vi "define_stimulus_shape.vi"(8 "error in":errorcluster, 10 "input cluster":T1={"base directory"=path "", "data directory"=path "", "active"=FALSE, "running"=FALSE, "pairing"=FALSE, "clean tubes"=FALSE, "animal ID"=0, "session ID"=0, "base temp"=0.0, "d wait min"=0, "d wait max"=0, "d timeout"=0, "d reward"=0, "idx stim"=0, "timeout win"=0, "lick win"=[], "stim type"=[], "stim dur"=[], "stim amp"=[], "stim freq"=[], "stim ramp"=[], "stim catch"=[], "square dur"=[50, 20, 10], "square delay"=[50, 20, 10], "square freq"=[], "square dc"=[50, 20, 10], "stim shape"=[], "square shape"=[]} {"stim ramp" min=1}) -> (0 "error out":errorcluster, 2 "output cluster":T1={"base directory"=path "", "data directory"=path "", "active"=FALSE, "running"=FALSE, "pairing"=FALSE, "clean tubes"=FALSE, "animal ID"=0, "session ID"=0, "base temp"=0.0, "d wait min"=0, "d wait max"=0, "d timeout"=0, "d reward"=0, "idx stim"=0, "timeout win"=0, "lick win"=[], "stim type"=[enum."sine", enum."square", enum."pulse"], "stim dur"=[500, 500, 1000], "stim amp"=[1.0, 1.0, 1.0], "stim freq"=[20, 20, 20], "stim ramp"=[100, 200, 200], "stim catch"=[], "square dur"=[50, 20, 10], "square delay"=[50, 20, 10], "square freq"=[], "square dc"=[50, 20, 10], "stim shape"=array3x1000[3000 elements], "square shape"=[]} {"stim ramp" min=1})   [LabVIEW 2016]
uses:
  Type Definitions/vars_settings.ctl
  Type Definitions/stim_type.ctl
  <vilib>/Analysis/1siggen.llb/Ramp Pattern.vi
  <vilib>/Analysis/1siggen.llb/Ramp Pattern by Samples.vi
  <vilib>/Utility/error.llb/Error Cluster From Error Code.vi
  <vilib>/Analysis/NI_AALBase.lvlib
panel:
  out "stim shape":dbl[][](graph)
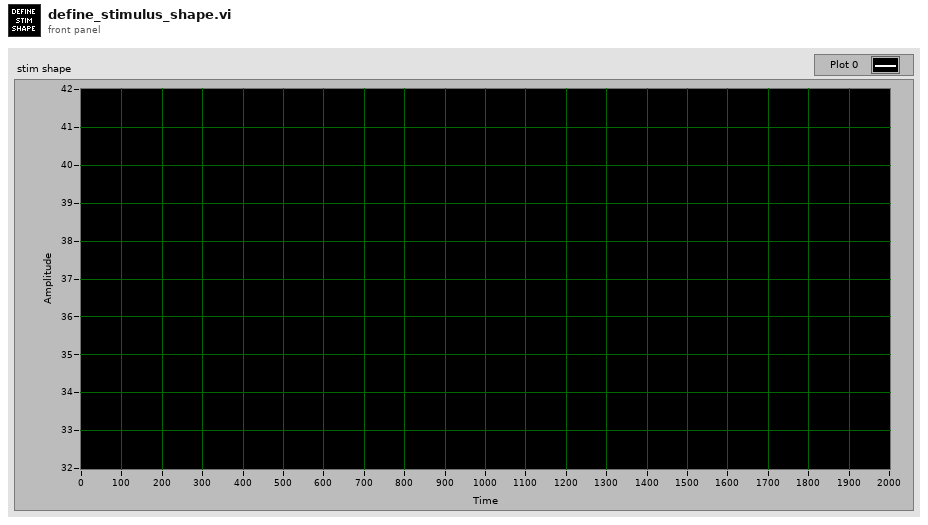
[diagram p1: front panel]
types:
  T1 = typedef "vars_settings.ctl" = cluster{"base directory":path, "data directory":path, "active":bool, "running":bool, "pairing":bool, "clean tubes":bool, "animal ID":u16, "session ID":u16, "base temp":dbl, "d wait min":u16, "d wait max":u16, "d timeout":u16, "d reward":u16, "idx stim":u16, "timeout win":u16, "lick win":i32[], "stim type":T2[], "stim dur":u16[], "stim amp":dbl[], "stim freq":u16[], "stim ramp":u16[], "stim catch":u8[], "square dur":u8[], "square delay":u8[], "square freq":u8[], "square dc":u8[], "stim shape":dbl[][], "square shape":bool[][]}
  T2 = typedef "stim_type.ctl" = enum16{"pulse", "vibration", "square", "sine"}
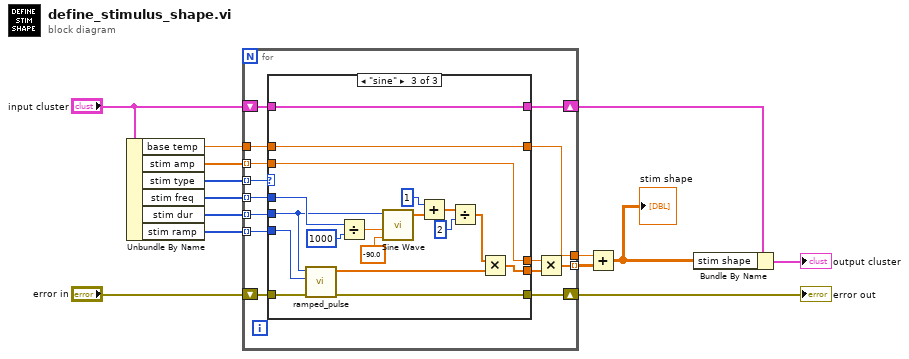
[diagram p0: block diagram]
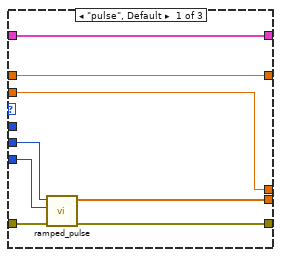
[diagram p2: hidden frame]
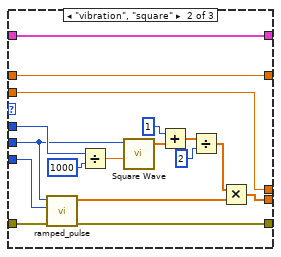
[diagram p3: hidden frame]
diagram:
  n1 = Unbundle By Name("input cluster") -> ("base temp"=w4:dbl, "stim amp"=w5:dbl[], "stim type"=w11:T2[], "stim freq"=w8:u16[], "stim dur"=w6:u16[], "stim ramp"=w7:u16[])
  n2 = for {
    tunnel: w11 -> [w25] mode=indexing
    shift-right: [w28] -> w14
    shift-left: "error in" -> [w27]
    shift-right: [w24] -> w9
    shift-left: "input cluster" -> [w26]
    tunnel: w8 -> [w23] mode=indexing
    tunnel: w6 -> [w22] mode=indexing
    tunnel: w7 -> [w21] mode=indexing
    tunnel: w5 -> [w20] mode=indexing
    tunnel: w4 -> [w19]
    tunnel: [w16] -> w3 mode=indexing
    tunnel: [w15] -> w2
    n3 = case shown="\"sine\"" w25 {
      tunnel: [w36 w53 w71] -> w28
      tunnel: w27 -> [w35 w52 w70]
      tunnel: w26 -> [w34 w51 w69]
      tunnel: [w34 w51 w69] -> w24
      tunnel: [w29 w42 w62] -> w18
      tunnel: w22 -> [w30 w40 w57]
      tunnel: w21 -> [w33 w39 w56]
      tunnel: w23 -> [_ w41 w58]
      tunnel: w20 -> [w32 w37 w54]
      tunnel: [w32 w37 w54] -> w17
      tunnel: [w31 w38 w55] -> w15
      tunnel: w19 -> [w31 w38 w55]
      frame "pulse", Default {
        n4 = call "ramped_pulse.vi"("error in"=w35, "d ramp"=w33, "d stim"=w30) -> ("error out"=w36:errorcluster, "output"=w29:dbl[])  [unwired: 7 in]
      }
      frame "vibration", "square" {
        n5 = call "ramped_pulse.vi"("error in"=w52, "d ramp"=w39, "d stim"=w40) -> ("error out"=w53:errorcluster, "output"=w43:dbl[])  [unwired: 7 in]
        n6 = Divide(x=w41, y=u16 1000) -> (x/y=w49:dbl)
        n7 = call <vilib>:"Square Wave.vi"("samples"=w40, "frequency"=w49) -> ("square wave"=w48:dbl[])  [unwired: 4 in, 2 out]
        n8 = Add(x=1, y=w48) -> (x+y=w46:dbl[])
        n9 = Divide(x=w46, y=2) -> (x/y=w44:dbl[])
        n10 = Multiply(x=w44, y=w43) -> (x*y=w42:dbl[])
      }
      frame "sine" {
        n11 = call "ramped_pulse.vi"("error in"=w70, "d ramp"=w56, "d stim"=w57) -> ("error out"=w71:errorcluster, "output"=w63:dbl[])  [unwired: 7 in]
        n12 = Divide(x=w58, y=u16 1000) -> (x/y=w60:dbl)
        n13 = call <vilib>:"Sine Wave.vi"("samples"=w57, "frequency"=w60, "phase in"=-90.0) -> ("sine wave"=w61:dbl[])  [unwired: 2 in, 2 out]
        n14 = Add(x=1, y=w61) -> (x+y=w66:dbl[])
        n15 = Divide(x=w66, y=2) -> (x/y=w64:dbl[])
        n16 = Multiply(x=w64, y=w63) -> (x*y=w62:dbl[])
      }
    }
    n17 = Multiply(x=w17, y=w18) -> (x*y=w16:dbl[])
  }
  "error out" <- w14
  n18 = Add(x=w2, y=w3) -> (x+y=w1:dbl[][])
  "stim shape" <- w1
  n19 = Bundle By Name(cluster=w9, "stim shape"=w1) -> (→"output cluster":T1)
